vi "okCFrontPanelDevices Get Flash Memory Layout.vi"(8 "error in (no error)":errorcluster, 11 "okTFlashLayout Refnum":refnum<k24>) -> (0 "error out":errorcluster, 2 "Flash Memory Layout":T1)   [LabVIEW 2019, in "okFrontPanelC#Wrapper.lvlib"]
uses:
  okFrontPanelC#Wrapper.lvlib
  C:/UCLA Thinkpad Google Drive/LabVIEW 2019 SP1/builds/SS2 Live Distribution/Opal Kelly/C# Wrapper/libFrontPanel-csharp.dll
  libFrontPanel-csharp.dll
  okTFlashLayoutStruct.ctl
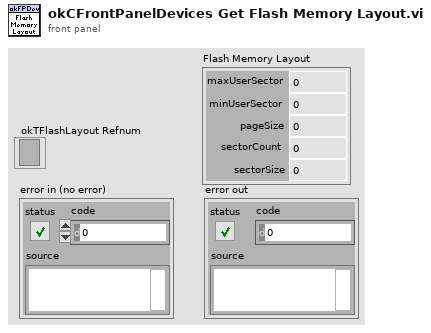
[diagram p1: front panel]
types:
  T1 = typedef "okFrontPanelC#Wrapper.lvlib/okTFlashLayoutStruct.ctl" = cluster{"maxUserSector":u32, "minUserSector":u32, "pageSize":u32, "sectorCount":u32, "sectorSize":u32}
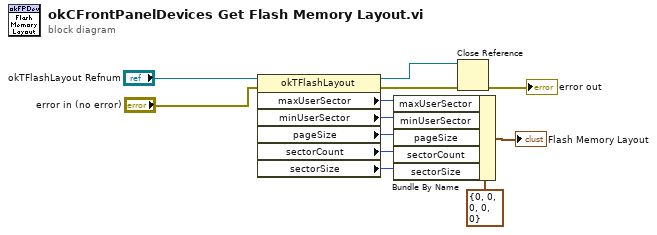
[diagram p0: block diagram]
diagram:
  n1 = property class="okTFlashLayout"(reference="okTFlashLayout Refnum", error in="error in (no error)") -> (reference out=w8:refnum<k24>, error out=w12:errorcluster, "maxUserSector"=w7:u32, "minUserSector"=w6:u32, "pageSize"=w5:u32, "sectorCount"=w4:u32, "sectorSize"=w3:u32)
  n2 = Bundle By Name(cluster=T1 {"maxUserSector"=0, "minUserSector"=0, "pageSize"=0, "sectorCount"=0, "sectorSize"=0} ("output cluster"), "maxUserSector"=w7, "minUserSector"=w6, "pageSize"=w5, "sectorCount"=w4, "sectorSize"=w3) -> (→"Flash Memory Layout":T1)
  n3 = Close Reference(reference=w8, error in (no error)=w12) -> (error out=→"error out":errorcluster)
